vi "queue_arrays.vi"() -> ()   [LabVIEW 2019]
uses:
  <vilib>/Analysis/1siggen.llb/General Aperiodic Triangle.vi
  <vilib>/Analysis/NI_AALBase.lvlib
panel:
  out "Waveform Graph":dbl[](graph)
  in  "stop":bool
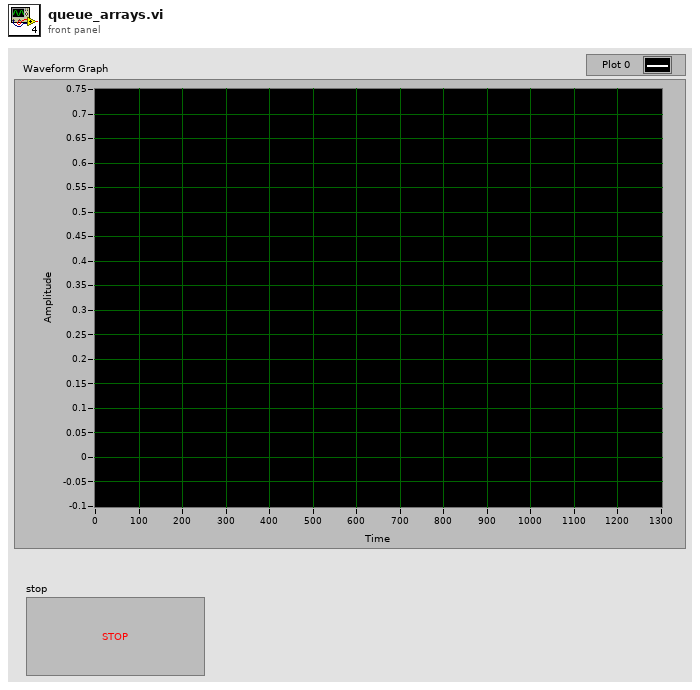
[diagram p1: front panel]
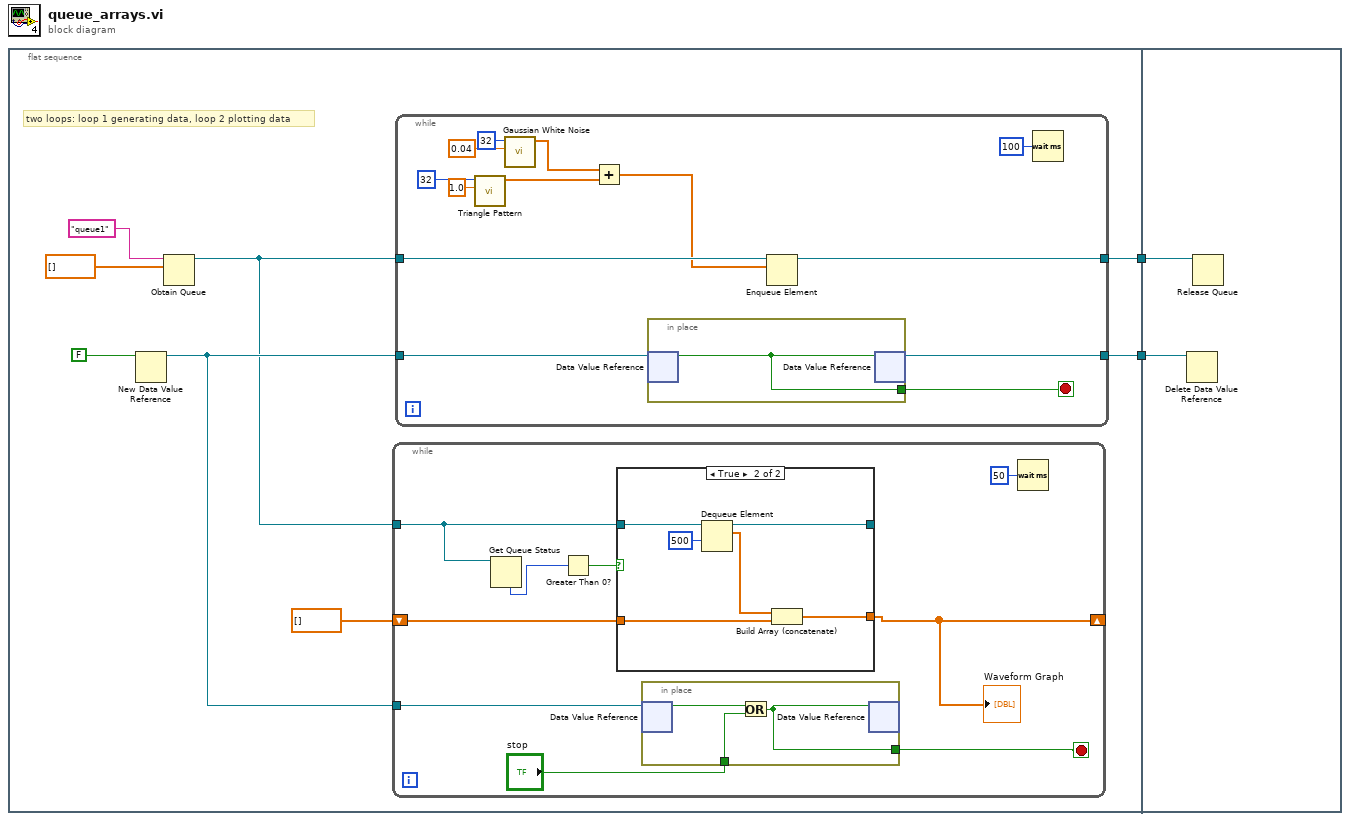
[diagram p0: block diagram]
diagram:
  n1 = flat-sequence {
    tunnel: [w4] -> w2
    tunnel: [w3] -> w1
    tunnel: w2 -> [w46]
    tunnel: w1 -> [w45]
    frame #0 {
      # "two loops: loop 1 generating data, loop 2 plotting data"
      n2 = New Data Value Reference(data value=FALSE) -> (data value reference=w9:refnum<data-value>)  [unwired: 1 in, 1 out]
      n3 = Obtain Queue(name (unnamed)="queue1", element data type=dbl[] []) -> (queue out=w6:refnum<queue>)  [unwired: 3 in, 2 out]
      n4 = while {
        tunnel: w9 -> [w18]
        tunnel: w6 -> [w15]
        shift-right: [w11] -> _
        shift-left: dbl[] [] -> [w12]
        stop <- w16 stop-if-true
        n5 = Get Queue Status(queue=w15) -> (# elements in queue=w14:i32)  [unwired: 2 in, 7 out]
        n6 = Greater Than 0?(x=w14) -> (x > 0?=w13:bool)
        n7 = case shown="True" w13 {
          tunnel: w15 -> [w21 w27]
          tunnel: [w21 w25] -> _
          tunnel: w12 -> [w20 w23]
          tunnel: [w20 w22] -> w11
          frame False {
          }
          frame True {
            n8 = Dequeue Element(queue=w27, timeout in ms (-1)=500) -> (queue out=w25:refnum<queue>, element=w24:dbl[])  [unwired: 1 in, 2 out]
            n9 = Build Array (concatenate)(w24, w23) -> (w22:dbl[])
          }
        }
        "Waveform Graph" <- w11
        n10 = in-place {
          in-place-border: "stop" -> [w29]
          in-place-border: [w28] -> w16
          n11 = in-place-dvr #1(w18) -> (w30:bool)  [unwired: 1 out]
          n12 = Or(x=w30, y=w29) -> (x .or. y?=w28:bool)
          n13 = in-place-dvr #1(w28) -> ()  [unwired: 2 out]
        }
        n14 = Wait (ms)(milliseconds to wait=u32 50) -> ()  [unwired: 1 out]
      }
      n15 = while {
        tunnel: w9 -> [w36]
        tunnel: w6 -> [w34]
        tunnel: [w32] -> w4
        tunnel: [w31] -> w3
        stop <- w35 stop-if-true
        n16 = call <vilib>:"Triangle Pattern.vi"("amplitude"=1.0, "samples"=32) -> ("Triangle Pattern"=w38:dbl[])  [unwired: 8 in, 1 out]
        n17 = call <vilib>:"Gaussian White Noise.vi"("standard deviation"=0.04, "samples"=32) -> ("Gaussian noise pattern"=w39:dbl[])  [unwired: 8 in, 1 out]
        n18 = Add(x=w39, y=w38) -> (x+y=w33:dbl[])
        n19 = in-place {
          in-place-border: [w44] -> w35
          n20 = in-place-dvr #2(w36) -> (w44:bool)  [unwired: 1 out]
          n21 = in-place-dvr #2(w44) -> (w31:refnum<data-value>)  [unwired: 1 out]
        }
        n22 = Enqueue Element(queue=w34, element=w33) -> (queue out=w32:refnum<queue>)  [unwired: 2 in, 2 out]
        n23 = Wait (ms)(milliseconds to wait=u32 100) -> ()  [unwired: 1 out]
      }
    }
    frame #1 {
      n24 = Delete Data Value Reference(data value reference=w45) -> ()  [unwired: 1 in, 2 out]
      n25 = Release Queue(queue=w46) -> ()  [unwired: 2 in, 3 out]
    }
  }
